vi "DO_Write.vi"(3 "error in (no error)":errorcluster, 4 "data in":u8[](array[numeric]), 5 "Task ID":u32) -> (0 "error out":errorcluster, 2 "Task ID":u32)   [LabVIEW 2015]
uses:
  Windows/System32/AdvLvDaq.dll
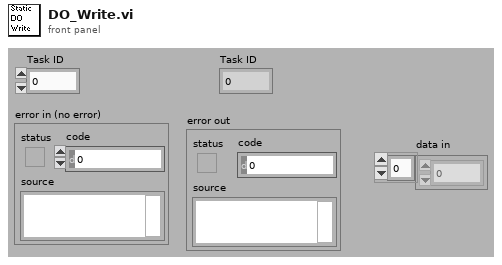
[diagram p1: front panel]
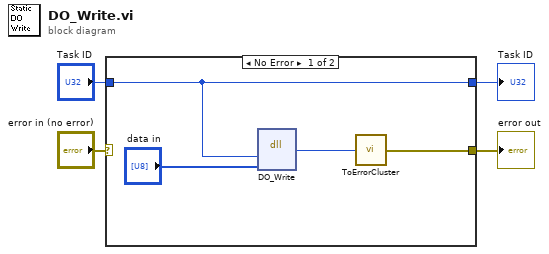
[diagram p0: block diagram]
diagram:
  n1 = case shown="No Error" "error in (no error)" {
    selector: "error in (no error)" -> [_ w10]
    tunnel: "Task ID" -> [w7 w9]
    tunnel: [w5 w10] -> w3
    tunnel: [w7 w9] -> w1
    frame No Error {
      n2 = dll-call lib="C:/Windows/System32/AdvLvDaq.dll" fn="DO_Write"("taskId"=w7, "data"="data in") -> ("return type"=w8:i32)  [unwired: 5 in, 2 out]
      n3 = call "ToErrorCluster.vi"("error code"=w8) -> ("error out"=w5:errorcluster)
    }
    frame Error {
    }
  }
  "error out" <- w3
  "Task ID" <- w1
